vi "Write Files.vi"(8 "error in (no error)":errorcluster, 11 "Masterv2 in":refnum<class "Masterv2.lvclass">) -> (0 "error out":errorcluster, 3 "Masterv2 out":refnum<class "Masterv2.lvclass">)   [LabVIEW 2014, in "Main Libraryv2.lvlib" / "Masterv2.lvclass"]
uses:
  Master/Masterv2.lvclass
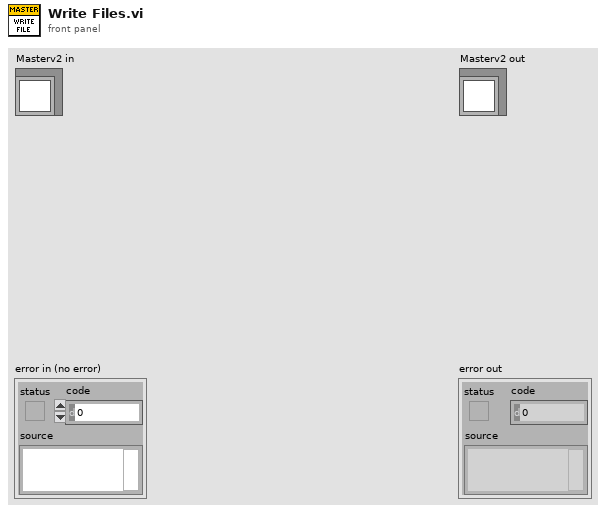
[diagram p1: front panel]
types:
  T1 = enum16{"open", "replace", "create", "open or create", "replace or create", "replace or create with confirmation"}
  T2 = cluster{"type string":i16[], "data string":string}
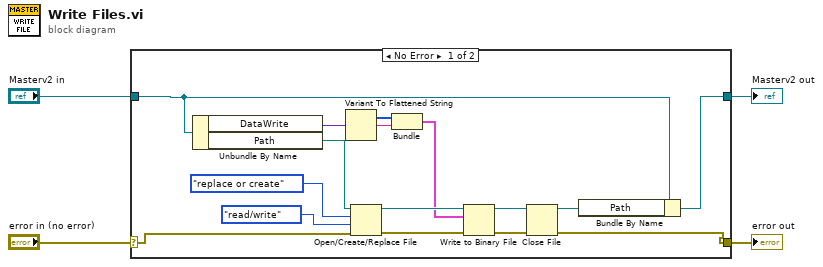
[diagram p0: block diagram]
diagram:
  n1 = case shown="No Error" "error in (no error)" {
    selector: "error in (no error)" -> [w8 w22]
    tunnel: [w7 w22] -> w3
    tunnel: [w5 w21] -> w1
    tunnel: "Masterv2 in" -> [w6 w21]
    frame No Error {
      n2 = Unbundle By Name(w6) -> ("DataWrite"=w10:variant, "Path"=w20:path)
      n3 = Variant To Flattened String(Variant=w10) -> (data string=w12:string, 1:w13:i16[])
      n4 = Open/Create/Replace File(file path (use dialog)=w20, error in=w8, operation (0:open)=T1."replace or create", access (0:read/write)=enum16{"read/write", "read-only", "write-only"}."read/write") -> (refnum out=w17:refnum<file>, error out=w16:errorcluster)  [unwired: 2 in, 1 out]
      n5 = Bundle("type string"=w13, "data string"=w12) -> (w11:T2)  [unwired: 1 in]
      n6 = Write to Binary File(file (use dialog)=w17, data=w11, error in=w16) -> (refnum out=w15:refnum<file>, error out=w14:errorcluster)  [unwired: 3 in, 1 out]
      n7 = Close File(refnum=w15, error in=w14) -> (path=w9:path, error out=w7:errorcluster)
      n8 = Bundle By Name(cluster=w6, "Path"=w9) -> (w5:refnum<class "Masterv2.lvclass">)
    }
    frame Error {
    }
  }
  "error out" <- w3
  "Masterv2 out" <- w1
